vi "POST Buffer.vi"(6 "timeout (10000)":i32=10000, 7 "output file":path=path "", 8 "error in (no error)":errorcluster, 9 "buffer":string, 10 "url":string, 11 "HTTP Client Advanced in":refnum<class "HTTP Client Advanced.lvclass">) -> (0 "error out":errorcluster, 1 "body":string, 2 "headers":string, 3 "HTTP Client Advanced out":refnum<class "HTTP Client Advanced.lvclass">)   [LabVIEW 2021, in "HTTP Client Advanced.lvclass"]
uses:
  HTTP Client Advanced.lvclass
  HTTP Client Advanced.lvclass/HTTP Client Advanced.ctl
  <vilib>/NI/Advanced HTTP Client/Session.lvclass
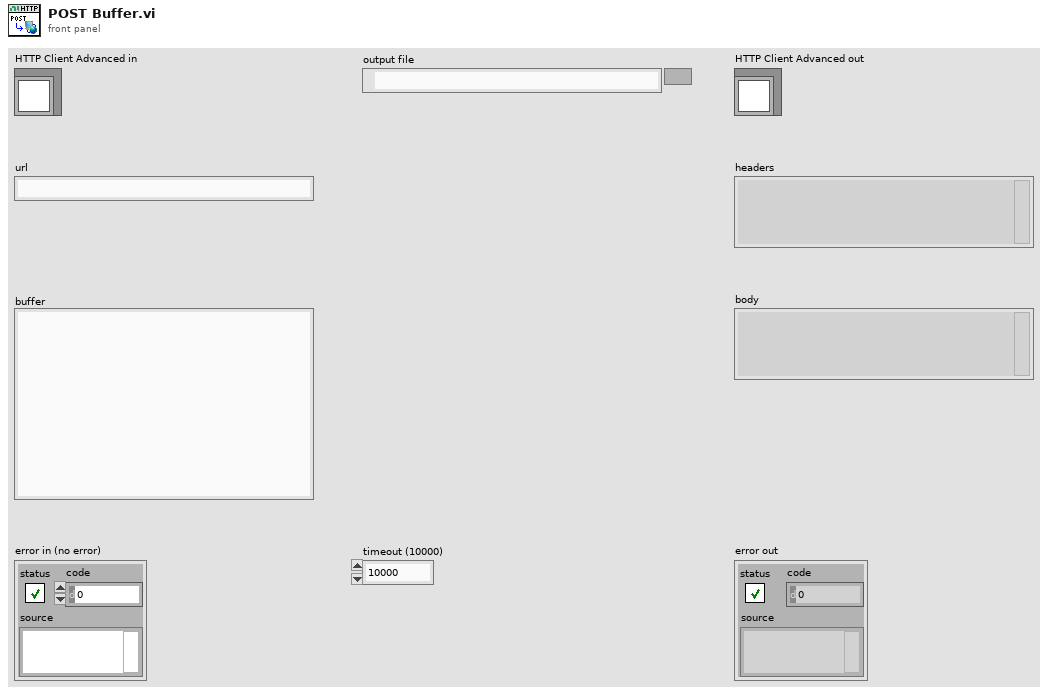
[diagram p1: front panel]
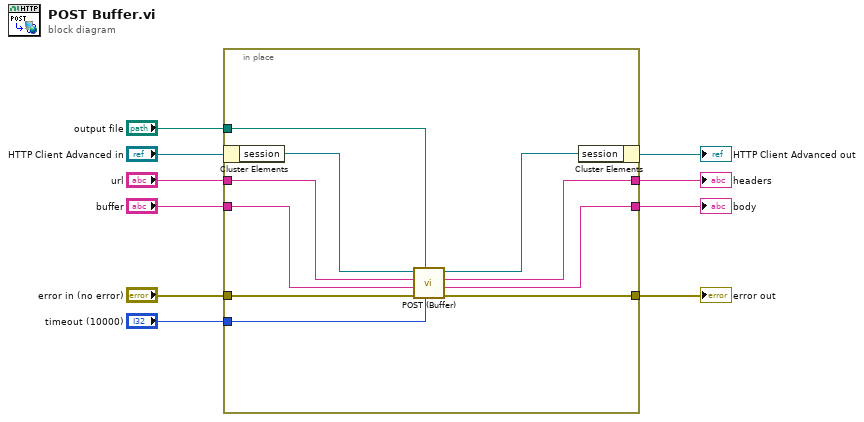
[diagram p0: block diagram]
diagram:
  n1 = in-place {
    in-place-border: "error in (no error)" -> [w18]
    in-place-border: [w17] -> w8
    in-place-border: "timeout (10000)" -> [w16]
    in-place-border: "output file" -> [w15]
    in-place-border: "url" -> [w14]
    in-place-border: "buffer" -> [w13]
    in-place-border: [w12] -> w3
    in-place-border: [w11] -> w2
    n2 = in-place-cluster #1("HTTP Client Advanced in") -> ("session"=w20:refnum<class "Session.lvclass">)
    n3 = call <vilib>:"POST (Buffer).vi"("timeout"=w16, "output file"=w15, "error in"=w18, "buffer"=w13, "url"=w14, "session in"=w20) -> ("error out"=w17:errorcluster, "body"=w11:string, "headers"=w12:string, "session out"=w19:refnum<class "Session.lvclass">)  [unwired: 1 in, 1 out]
    n4 = in-place-cluster #1("session"=w19) -> (→"HTTP Client Advanced out":refnum<class "HTTP Client Advanced.lvclass">)
  }
  "error out" <- w8
  "headers" <- w3
  "body" <- w2
